vi "Update Edit UI Values.vi"(8 "error in":errorcluster, 10 "Editable Nodes":T1(array[cluster]), 11 "VI Ref":refnum<vi>) -> (0 "error out":errorcluster)   [LabVIEW 2025]
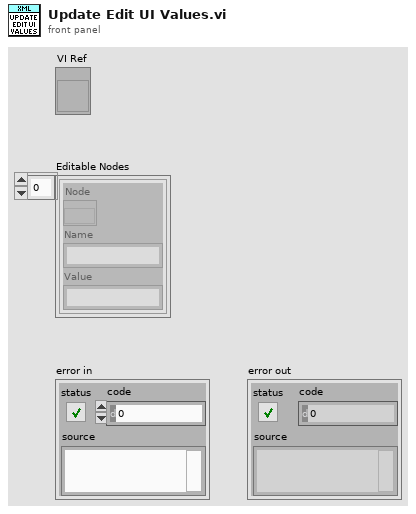
[diagram p1: front panel]
types:
  T1 = cluster{"Node":refnum<k20>, "Name":string, "Value":string}[]
  T2 = cluster{"Node":refnum<k20>, "Name":string, "Value":string}
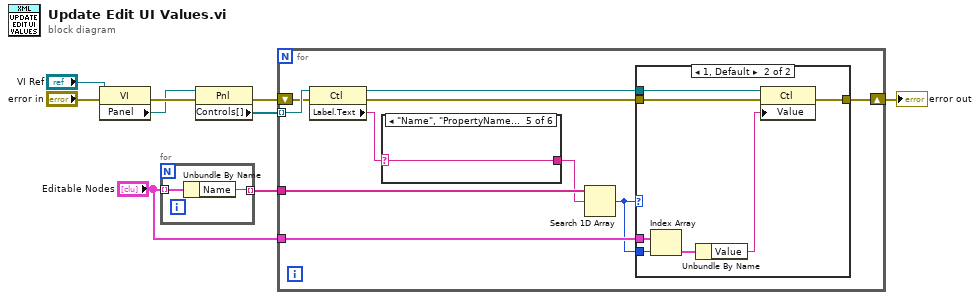
[diagram p0: block diagram]
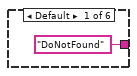
[diagram p3: hidden frame]
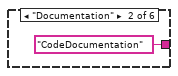
[diagram p4: hidden frame]
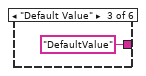
[diagram p5: hidden frame]
diagram:
  n1 = property class="VI"(reference="VI Ref", error in="error in") -> (error out=w8:errorcluster, "Panel"=w4:refnum<vi>)  [unwired: 1 out]
  n2 = for {
    tunnel: "Editable Nodes" -> [w11] mode=indexing
    tunnel: [w10] -> w2 mode=indexing
    n3 = Unbundle By Name(w11) -> ("Name"=w10:string)
  }
  n4 = property class="Pnl"(reference=w4, error in=w8) -> (error out=w5:errorcluster, "Controls[]"=w9:refnum<vi>[])  [unwired: 1 out]
  n5 = for {
    tunnel: w9 -> [w21] mode=indexing
    shift-right: [w13] -> w3
    shift-left: w5 -> [w20]
    tunnel: w2 -> [w18]
    tunnel: "Editable Nodes" -> [w16]
    n6 = property class="Ctl"(reference=w21, error in=w20) -> (reference out=w15:refnum<vi>, error out=w14:errorcluster, "Label.Text"=w19:string)
    n7 = case shown="\"Name\", \"PropertyName\"" w19 {
      selector: w19 -> [_ _ _ w33 w34 w35]
      tunnel: ["DoNotFound" ("element") "CodeDocumentation" ("element") "DefaultValue" ("element") w33 w34 w35] -> w17
      frame Default {
      }
      frame "Documentation" {
      }
      frame "Default Value" {
      }
      frame "Faultable", "Scalable", "Type", "Units" {
      }
      frame "Name", "PropertyName" {
      }
      frame "DataType", "GroupName", "TypeName" {
      }
    }
    n8 = Search 1D Array(1D array=w18, element=w17) -> (index of element=w12:i32)  [unwired: 1 in]
    n9 = case shown="1, Default" w12 {
      tunnel: w12 -> [_ w29]
      tunnel: w16 -> [_ w28]
      tunnel: w15 -> [_ w26]
      tunnel: w14 -> [w22 w24]
      tunnel: [w22 w23] -> w13
      frame -1 {
      }
      frame 1, Default {
        n10 = Index Array(array=w28, index=w29) -> (element=w27:T2)
        n11 = Unbundle By Name(w27) -> ("Value"=w25:string)
        n12 = property class="Ctl"(reference=w26, error in=w24, "Value"=w25) -> (error out=w23:errorcluster)  [unwired: 1 out]
      }
    }
  }
  "error out" <- w3
